vi "CL3IF_LightControl.vi"(8 "error in":errorcluster {"code" format="%x"}, 10 "onOff":bool, 11 "deviceId":i32) -> (0 "error out":errorcluster {"code" format="%x"})   [LabVIEW 2020, in "Keyence CL-3000.lvlib"]
doc: "This function turns on or turns off the measurement light."
uses:
  Keyence CL-3000.lvlib
  Private/enums/Function Name.ctl
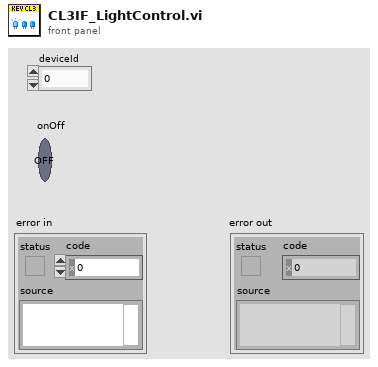
[diagram p1: front panel]
types:
  T1 = typedef "Keyence CL-3000.lvlib/Function Name.ctl" = enum16{"Initialize", "Close", "CL3IF_GetMeasurementData", "CL3IF_GetTrendIndex", "CL3IF_GetTrendData", "CL3IF_GetStorageIndex", "CL3IF_GetStorageData", "CL3IF_AutoZeroMulti", "CL3IF_AutoZeroGroup", "CL3IF_TimingMulti", "CL3IF_TimingGroup", "CL3IF_ResetMulti", "CL3IF_ResetGroup", "CL3IF_LightControl", "CL3IF_MeasurementControl", "CL3IF_SwitchProgram", "CL3IF_GetProgramNo", "CL3IF_StartStorage", "CL3IF_StopStorage", "CL3IF_ClearStorageData", "CL3IF_GetPulseCount", "CL3IF_ResetPulseCount", "CL3IF_GetLightWaveform"}
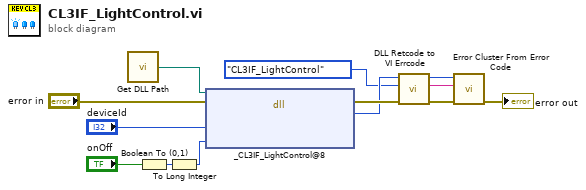
[diagram p0: block diagram]
diagram:
  n1 = call "Get DLL Path.vi"() -> ("DLL Path"=w7:path)  [unwired: 1 in]
  n2 = Boolean To (0,1)(Boolean="onOff") -> (0, 1=w10:i16)
  n3 = To Long Integer(number=w10) -> (32bit integer=w3:i32)
  n4 = dll-call lib="C:/Program Files (x86)/National Instruments/LabVIEW 2018/instr.lib/Keyence CL-3000/CL3_IF.dll" fn="_CL3IF_LightControl@8"(path in=w7, error in="error in", "deviceId"="deviceId", "onOff"=w3) -> (error out=w6:errorcluster, "RC"=w5:i32)  [unwired: 3 in, 1 out]
  n5 = call "DLL Retcode to VI Errcode.vi"("error in (no error)"=w6, "Function Name"=Function_Name."CL3IF_LightControl", "DLL Retcode"=w5) -> ("error out"=w13:errorcluster, "ErrorMessage"=w2:string, "VI Errcode"=w12:i32)  [unwired: 6 in]
  n6 = call <vilib>:"Error Cluster From Error Code.vi"("error in (no error)"=w13, "error message (\"\")"=w2, "error code (0)"=w12) -> ("error out"=→"error out":errorcluster)  [unwired: 6 in]
